vi "SQL.vi"(8 "error in (no error)":errorcluster, 11 "SQL Statement in":refnum<class "SQL Statement.lvclass">) -> (0 "error out":errorcluster, 2 "SQL":string, 3 "SQL Statement out":refnum<class "SQL Statement.lvclass">)   [LabVIEW 2023, in "SQLite.lvlib" / "SQL Statement.lvclass"]
doc: "Returns the text of the SQL for this prepared statement."
uses:
  SQL Statement.lvclass
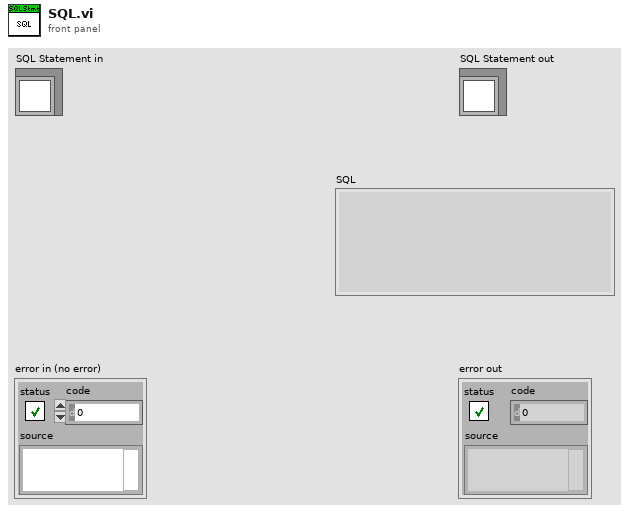
[diagram p1: front panel]
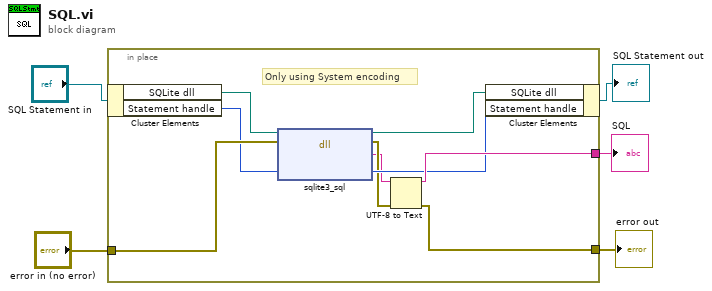
[diagram p0: block diagram]
diagram:
  n1 = in-place {
    in-place-border: "error in (no error)" -> [w14]
    in-place-border: [w13] -> w4
    in-place-border: [w12] -> w3
    # "Only using System encoding"
    n2 = in-place-cluster #1("SQL Statement in") -> ("SQLite dll"=w11:path, "Statement handle"=w10:u64)
    n3 = dll-call lib="C:/Users/Public/SSDC/SSDC-GenAppMainD2/Project/SourceCode/sqlite3x*.*" fn="sqlite3_sql"(path in=w11, error in=w14, "Statement"=w10) -> (path out=w8:path, error out=w7:errorcluster, "SQL"=w6:string, "Statement"=w9:u64)  [unwired: 1 in]
    n4 = UTF-8 to Text(8:w7, 11:w6) -> (0:w13:errorcluster, 3:w12:string)  [unwired: 1 in]
    n5 = in-place-cluster #1("SQLite dll"=w8, "Statement handle"=w9) -> (→"SQL Statement out":refnum<class "SQL Statement.lvclass">)
  }
  "error out" <- w4
  "SQL" <- w3
